vi "DrivePath.vi"() -> ()   [LabVIEW 2018]
uses:
  Dawgma Programming Library/Controls/PurePursuit/PathFileData.ctl
  Dawgma Programming Library/Controls/PurePursuit/RobotNeededPathData.ctl
  Framework/Robot Global Data.vi
panel:
  in  "PathFileName":string
  in  "Index":dbl
  in  "NoWait":bool
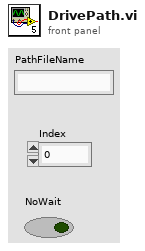
[diagram p1: front panel]
types:
  T1 = typedef "PathFileData.ctl" = cluster{"RobotNeeded":T2, "Meta":cluster{"Path (px)":cluster{i32, i32}[], "RobotWidth":dbl, "RobotLength":dbl, "CenterOfRotYOffset":dbl, "Roundedness":dbl, "StartingPositionPreset":u32}}
  T2 = typedef "RobotNeededPathData.ctl" = cluster{"Path":cluster{dbl, dbl}[], "MaxVel":dbl, "MaxAccel":dbl, "Backwards?":bool, "PointSpacing":dbl, "LookaheadDist":dbl, "Speed/Curve":dbl, "SlowDistanceAtEnd":dbl, "SlowSpeed":dbl, "MaxDeAccel":dbl}
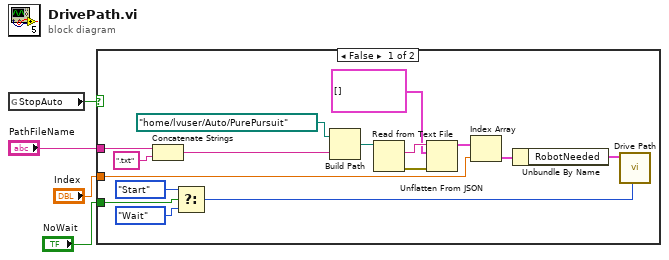
[diagram p0: block diagram]
diagram:
  n1 = global read "Robot Global Data.vi" "StopAuto"() -> (w4:bool)
  n2 = case shown="False" w4 {
    tunnel: "Index" -> [w11 _]
    tunnel: "NoWait" -> [w5 _]
    tunnel: "PathFileName" -> [w20 _]
    frame False {
      n3 = Concatenate Strings(w20, ".txt" ("string")) -> (w18:string)
      n4 = Select(t=enum16{"Start", "Wait"}."Start" ("Synchronization"), s=w5, f=enum16{"Start", "Wait"}."Wait" ("Synchronization")) -> (s? t:f=w6:enum16{"Start", "Wait"})
      n5 = Build Path(base path=path "/home/lvuser/Auto/PurePursuit", name or relative path=w18) -> (appended path=w16:path)
      n6 = Read from Text File(file (use dialog)=w16) -> (text=w14:string, error out=w15:errorcluster)  [unwired: 3 in, 2 out]
      n7 = Unflatten From JSON(JSON string=w14, type and defaults=T1[] [], error in (no error)=w15) -> (value=w12:T1[])  [unwired: 4 in, 1 out]
      n8 = Index Array(array=w12, index=w11) -> (element=w10:T1)
      n9 = Unbundle By Name(w10) -> ("RobotNeeded"=w9:T2)
      n10 = call "Drive Path.vi"("Synchronication"=w6, "RobotNeededPathData"=w9) -> ()  [unwired: 9 in, 1 out]
    }
    frame True {
    }
  }
